vi "To File (Path).vi"(5 "access (0:read/write)":enum16{"read/write", "read-only", "write-only"}(ring), 6 "Pretty Print?":bool=TRUE, 7 "enable LabVIEW extensions? (T)":bool=TRUE, 8 "error in (no error)":errorcluster, 9 "operation (0:open)":T1(ring), 10 "JSON Value in":refnum<class "JSON Value.lvclass">, 11 "file path":path) -> (0 "error out":errorcluster)   [LabVIEW 2016, in "JSON Value.lvclass"]
doc: "Saves a JSON instance's data to the given file."
uses:
  JSON Value.lvclass
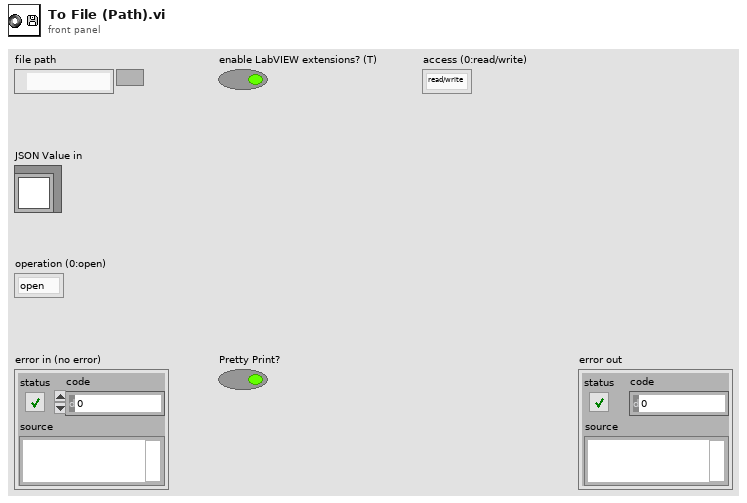
[diagram p1: front panel]
types:
  T1 = enum16{"open", "replace", "create", "open or create", "replace or create", "replace or create with confirmation"}
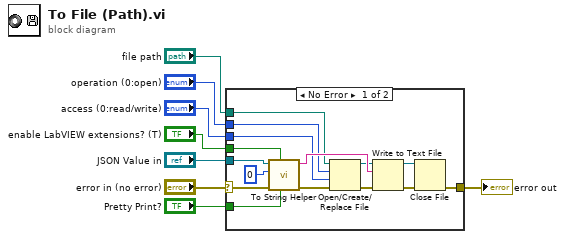
[diagram p0: block diagram]
diagram:
  n1 = case shown="No Error" "error in (no error)" {
    selector: "error in (no error)" -> [w18 w24]
    tunnel: "JSON Value in" -> [w23 _]
    tunnel: "file path" -> [w16 _]
    tunnel: [w13 w24] -> w5
    tunnel: "operation (0:open)" -> [w15 _]
    tunnel: "access (0:read/write)" -> [w14 _]
    tunnel: "Pretty Print?" -> [w10 _]
    tunnel: "enable LabVIEW extensions? (T)" -> [w11 _]
    frame No Error {
      n2 = call "To String Helper.vi"("pretty print? (T)"=w10, "enable LabVIEW extensions? (T)"=w11, "error in (no error)"=w18, "indent"=0, "JSON Value in"=w23) -> ("error out"=w12:errorcluster, "String"=w22:string)  [unwired: 5 in]
      n3 = Open/Create/Replace File(file path (use dialog)=w16, error in=w12, operation (0:open)=w15, access (0:read/write)=w14) -> (refnum out=w19:refnum<file>, error out=w17:errorcluster)  [unwired: 2 in, 1 out]
      n4 = Write to Text File(file (use dialog)=w19, text=w22, error in=w17) -> (refnum out=w20:refnum<file>, error out=w21:errorcluster)  [unwired: 1 in, 1 out]
      n5 = Close File(refnum=w20, error in=w21) -> (error out=w13:errorcluster)  [unwired: 1 out]
    }
    frame Error {
    }
  }
  "error out" <- w5
